vi "RunTest.vi"(8 "error in (no error)":errorcluster, 11 "Prueba10 in":refnum<class "Prueba10.lvclass">) -> (0 "error out":errorcluster, 2 "resultado":string, 3 "Prueba10 out":refnum<class "Prueba10.lvclass">)   [LabVIEW 2019, in "Prueba10.lvclass"]
uses:
  Prueba10.lvclass
  Prueba04/Control/Slide.ctl
  Prueba10.lvclass/Prueba10.ctl
  ClusterGEN.ctl
  <vilib>/Utility/error.llb/DialogType.ctl
  QMH/Message Queue/Enqueue Message (Single).vi
  <vilib>/Utility/error.llb/Error Cluster From Error Code.vi
  <vilib>/ErrorRing/Error Ring.xnode
  <vilib>/Utility/miscctls.llb/LVRowAndColumnTypeDef.ctl
  Prueba/Prueba.lvclass
  Controles/EstadosP10.ctl
  Controles/MessageP10.ctl
  QMH/User Event - Stop/User Event - Stop.lvlib
  QMH/Message Queue/Message Queue.lvlib
  Prueba04/Prueba04.lvclass
panel:
  out "Pict Ring 2":u16(ring)
  out "Pict Ring 3":u16(ring)
  out "cumple_no_cumple":bool
  out "Vref":dbl
  in  "Tab":enum32{"Page 1", "Page 2"}(tab)
  out "NivMaxMenosSens":dbl
  out "NivelRMSensayo":dbl
  out "frecuencia1":dbl
  in  "guardar_Vref":bool
  in  "generar1":bool
  in  "AjusteAmp":T1=40.0 caption="Ajuste de amplitud [mV]" scale=0.0..20000.0
  out "voltMon1":dbl format="%#.1f"
  out "frecMon1":dbl format="%#.1f"
  in  "seguir":bool
  out "Pict Ring 4":u16(ring)
  out "Pict Ring":u16(ring)
  in  "Tabla2":string[][](table)
  out "saltoMon":dbl format="%#.1f"
  in  "generar2":bool
  in  "resta":bool
  in  "suma":bool
  in  "salto":dbl(knob)=0.5 min=0.1 max=0.5 scale=0.1..0.5
  in  "semiciclo":dbl(knob)=1.0 min=1.0 max=2.0 scale=1.0..2.0
  in  "Tabla1":string[][](table)
  in  "salir":bool
  out "cumple":bool
  out "no_cumple":bool
  out "voltMon2":dbl format="%#.1f"
  out "frecMon2":dbl format="%#.1f"
  # "Selección de Señal de referencia 8000 Hz"
  # "Elección Señal de Referencia\nsegún marca y modelo de sonómetro"
  # "Nivel RMS para Ensayo"
  # "Nivel Máximo Rango \nMenos Sensible"
  # "Frecuencia"
  # "Monitoreo"
  # "Frecuencia"
  # "Hz"
  # "Voltaje"
  # "mV"
  # "10. Indicación de sobrecarga. IEC 61672-3: 2006 Cláusula 18"
  # "Tabla Resultados"
  # "Selección de Saltos"
  # "Selección Orientación Semiciclo"
  # "Cumple"
  # "No Cumple"
  # "10. Indicación de sobrecarga. IEC 61672-3: 2006 Cláusula 18"
  # "Monitoreo"
  # "Frecuencia"
  # "Hz"
  # "Voltaje"
  # "mV"
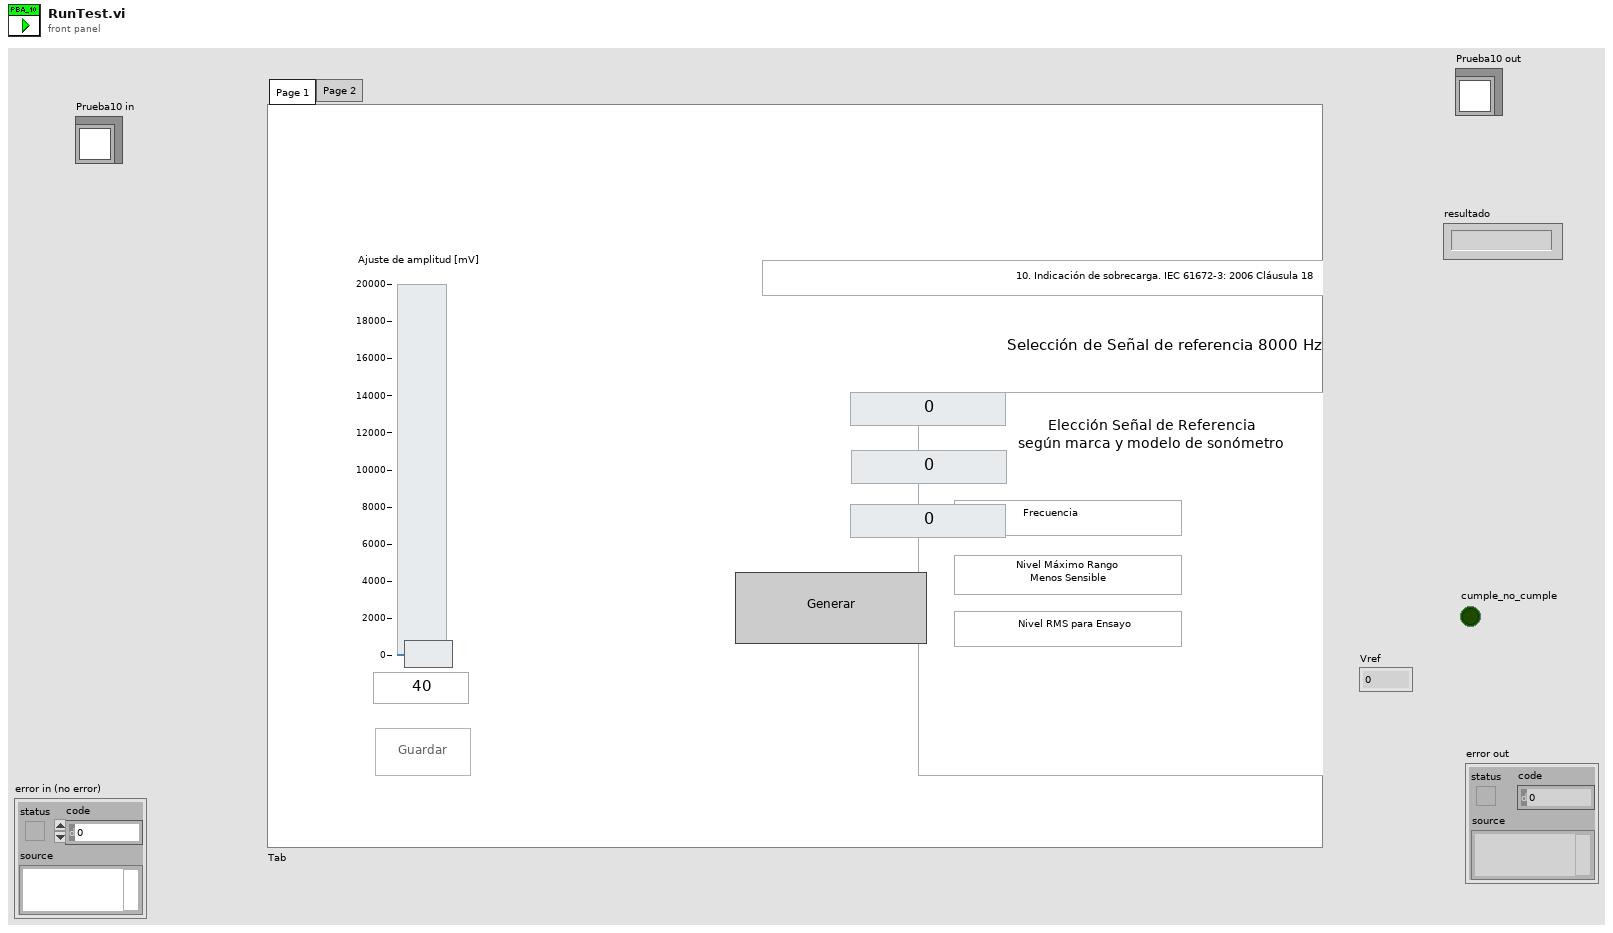
[diagram p1: front panel]
types:
  T1 = typedef "Prueba04.lvclass/Slide.ctl" = dbl
  T2 = typedef "LVRowAndColumnTypeDef.ctl" = cluster{"Row":i32, "Column":i32}
  T3 = typedef "Message Queue.lvlib/All Message Queues.ctl" = cluster{"MHL":refnum<queue>, "Inst_CNT90":refnum<queue>, "Inst_DS360":refnum<queue>, "Inst_Keithley2002":refnum<queue>, "Inst_DAQ":refnum<queue>, "BD":refnum<queue>, "Pistofono":refnum<queue>, "Nexus":refnum<queue>}
  T4 = enum32{"Page 1", "Page 2", "Page 3", "Page 4", "Page 5", "Page 6", "Page 7"}
  T5 = typedef "Prueba10.lvclass/ClusterGEN.ctl" = cluster{"frec":dbl, "amp":dbl}
  T6 = typedef "Prueba10.lvclass/EstadosP10.ctl" = enum16{"DetieneInstrumentos", "InicializarInstrumentos", "LeerArchivoConfiguracion", "Error", "inicio", "configurarTabla", "FrecAmp1", "FrecAmp2", "FrecAmp3", "suma_resta", "calcularVref", "iniciarGEN", "iniciarGEN_2", "reset-NivRefEnsayo", "guardaVref", "monitoreo", "monitoreo_2", "ingresaMediciones", "guardarMediciones", "detenerGEN", "cumplimiento", "listo_evaluar", "evaluar", "final", "salir"}
  T7 = typedef "Prueba10.lvclass/MessageP10.ctl" = cluster{"Estados":T6, "Data":variant}
  T8 = enum8{"Enabled", "Disabled", "Disabled and Grayed Out"}
  T9 = cluster{"ControlName":string, "ControlReference":refnum<vi>}[]
  T10 = typedef "DialogType.ctl" = u16
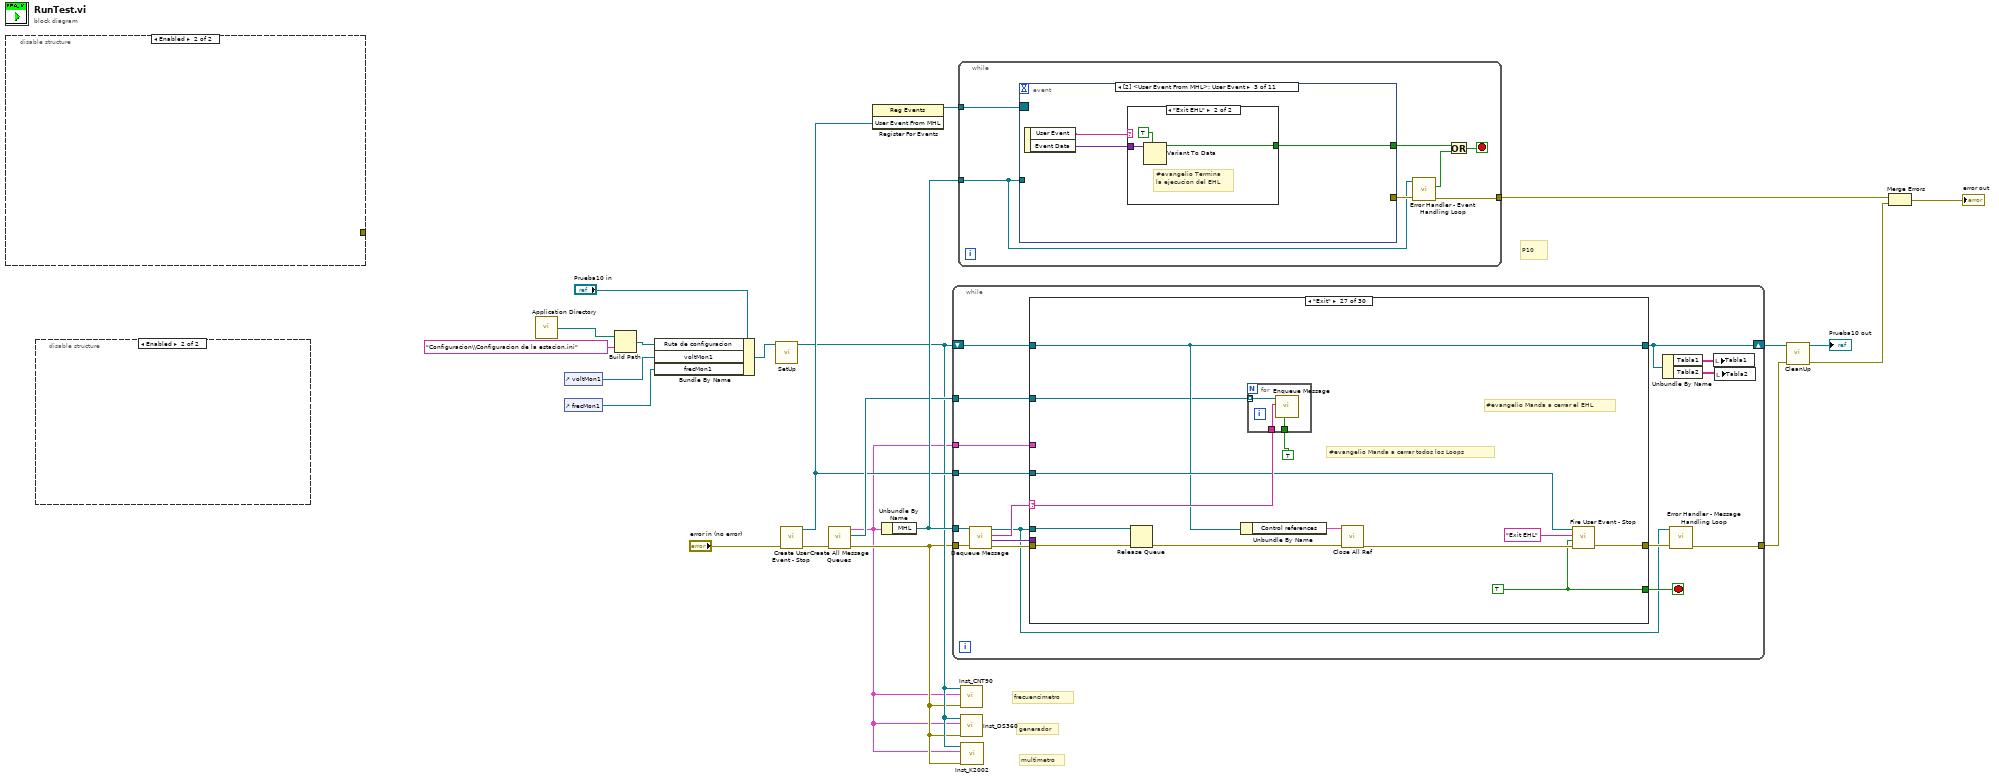
[diagram p0: block diagram]
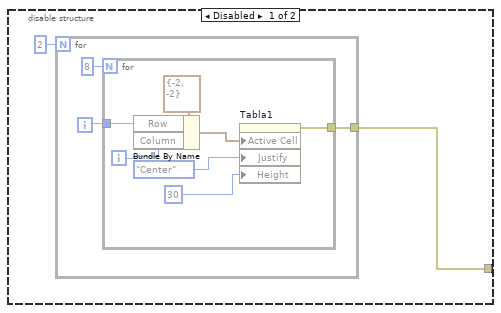
[diagram p2: hidden frame]
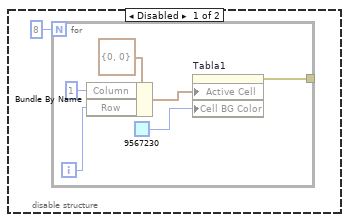
[diagram p3: hidden frame]
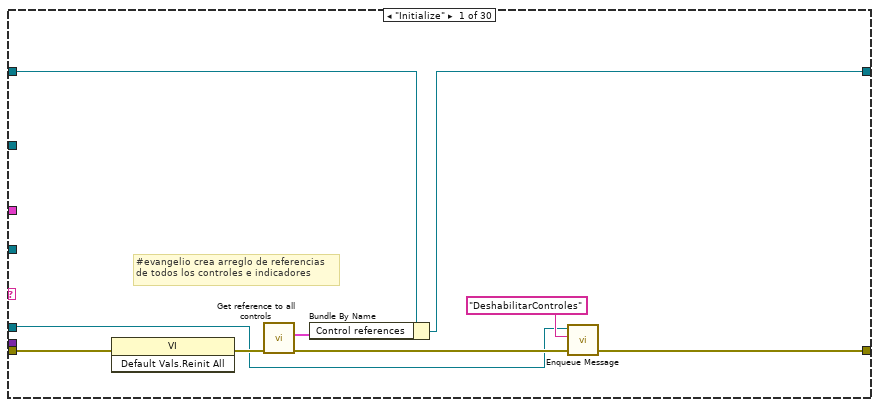
[diagram p4: hidden frame]
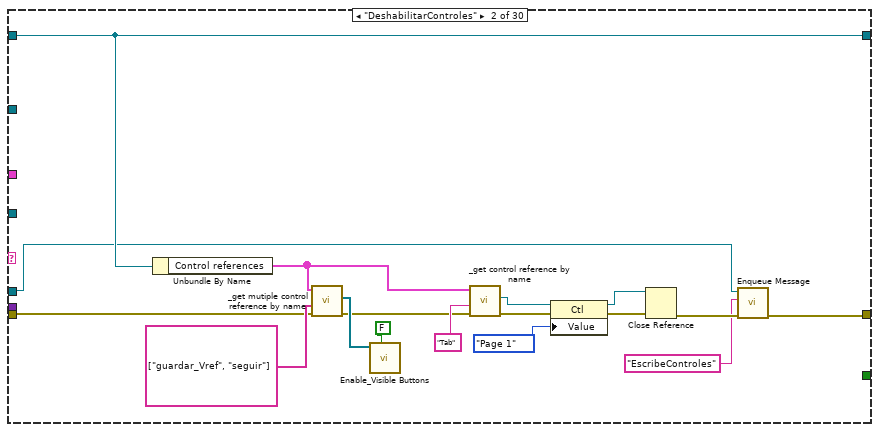
[diagram p5: hidden frame]
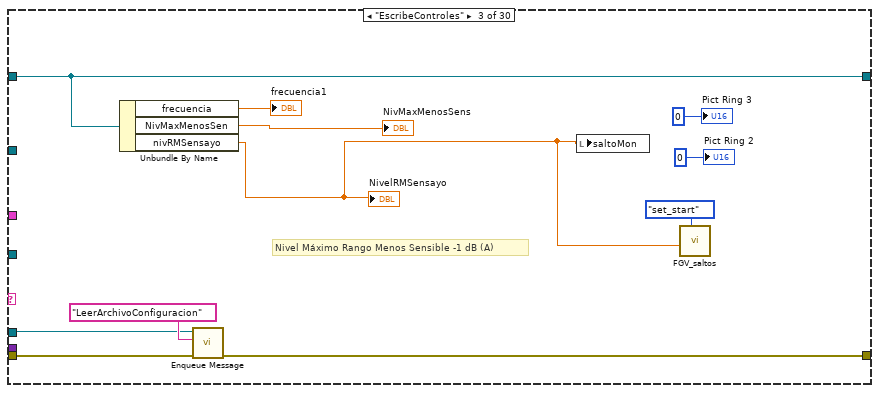
[diagram p6: hidden frame]
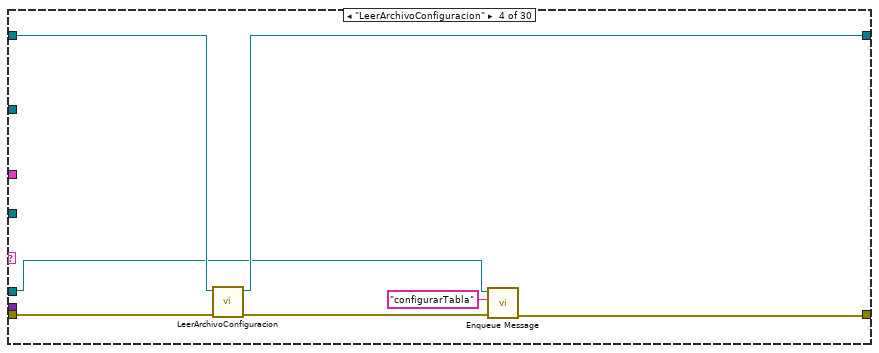
[diagram p7: hidden frame]
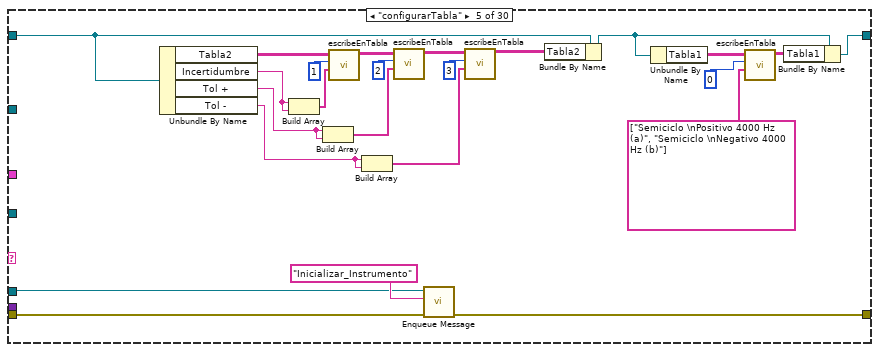
[diagram p8: hidden frame]
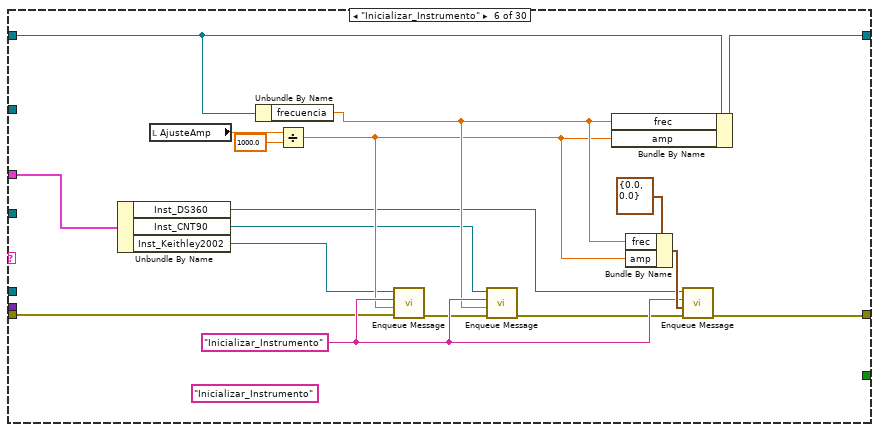
[diagram p9: hidden frame]
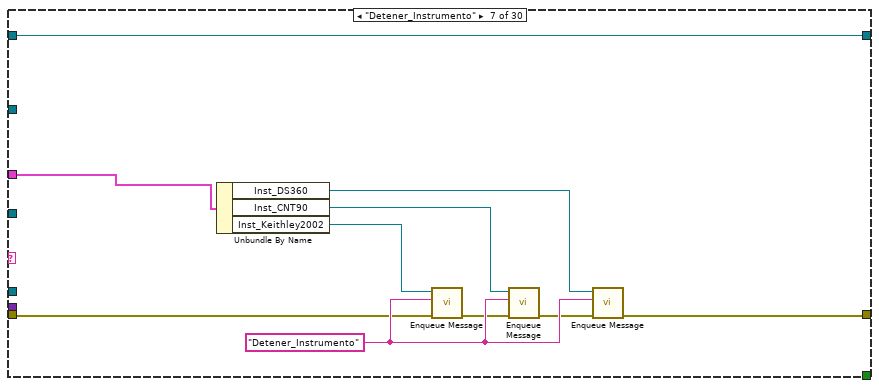
[diagram p10: hidden frame]
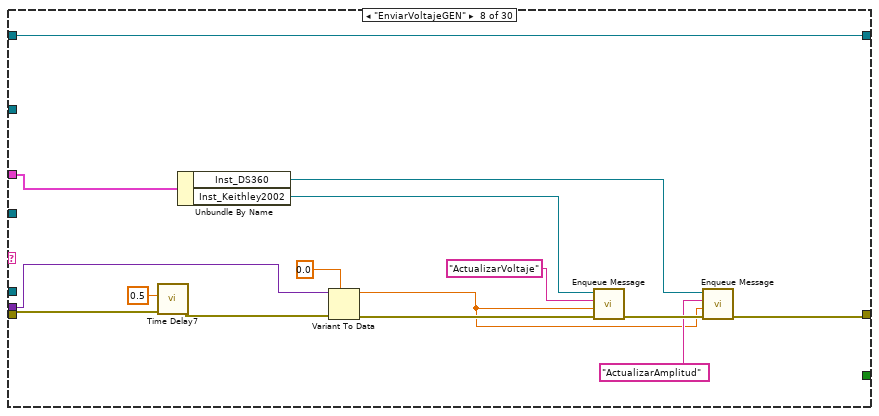
[diagram p11: hidden frame]
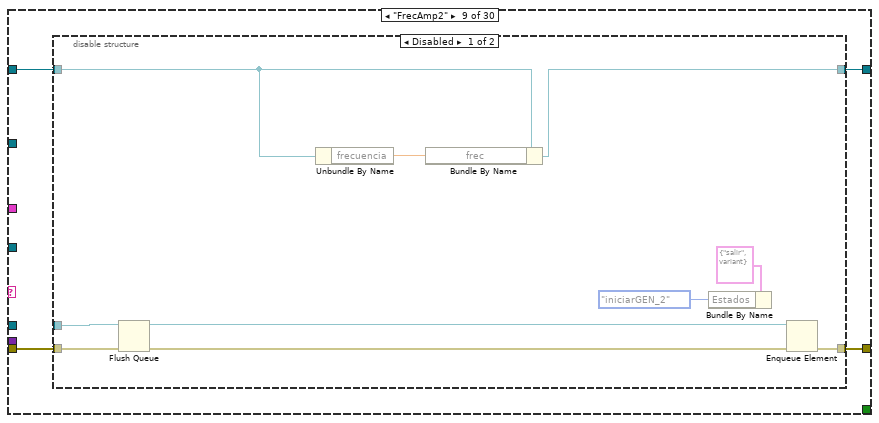
[diagram p12: hidden frame]
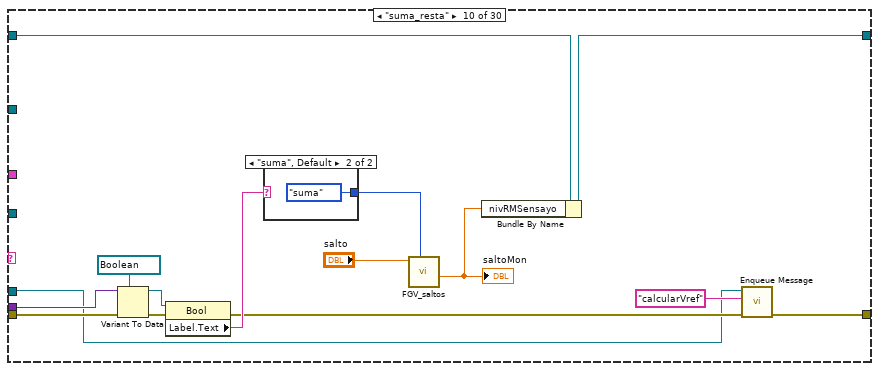
[diagram p14: hidden frame]
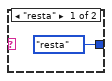
[diagram p15: hidden frame]
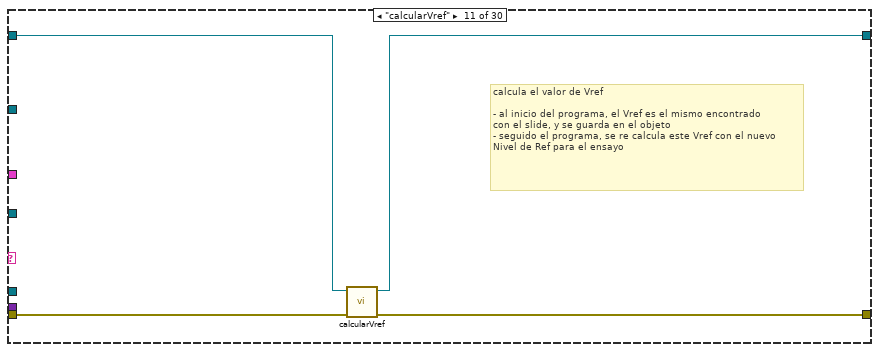
[diagram p16: hidden frame]
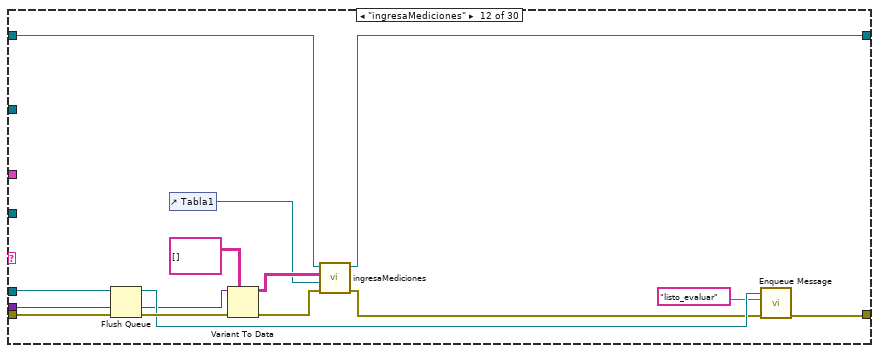
[diagram p17: hidden frame]
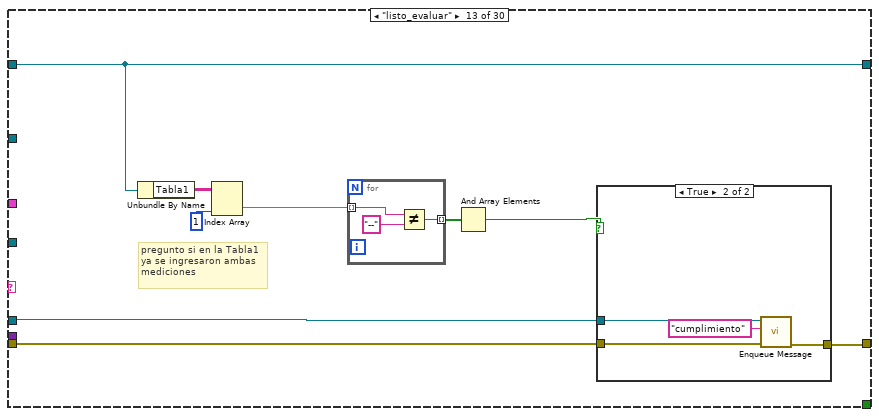
[diagram p18: hidden frame]
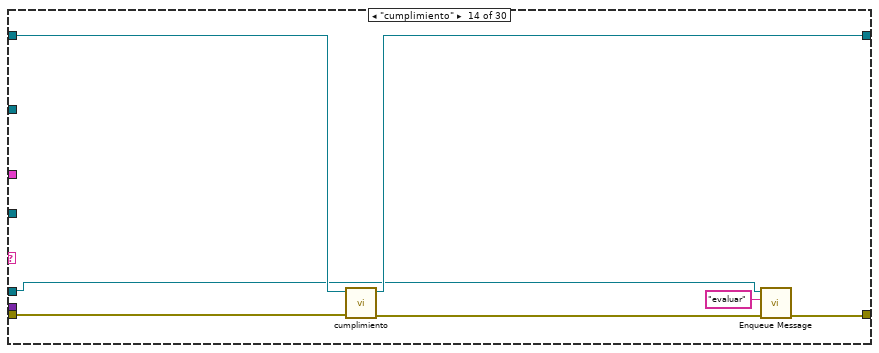
[diagram p20: hidden frame]
diagram:
  # "multimetro"
  # "generador"
  # "frecuencimetro"
  # "P10"
  n1 = disable-structure shown="Enabled" {
    disable-tunnel: [w24 _] -> _
    frame Disabled {
      n2 = for {
        N: 2 -> [_]
        tunnel: [w27] -> w24
        i -> [w26]
        n3 = for {
          N: 8 -> [_]
          tunnel: [w32] -> w27
          tunnel: w26 -> [w29]
          i -> [w28]
          n4 = Bundle By Name(cluster=T2 {"Row"=-2, "Column"=-2} ("Active Cell:Active Cell"), "Row"=w29, "Column"=w28) -> (w30:T2)
          n5 = property on="Tabla1" class="Tbl (strict)"("Active Cell"=w30, "Justify"=enum16{"Left", "Center", "Right"}."Center" ("Active Cell:Cell Justification"), "Height"=u32 30 ("Active Cell:Cell Font:Size")) -> (error out=w32:errorcluster)  [unwired: 2 in, 1 out]
        }
      }
    }
    frame Enabled {
    }
  }
  n6 = disable-structure shown="Enabled" {
    frame Disabled {
      n7 = for {
        N: 8 -> [_]
        tunnel: [w37] -> _
        i -> [w36]
        n8 = Bundle By Name(cluster=T2 {"Row"=0, "Column"=0} ("Active Cell:Active Cell"), "Column"=1, "Row"=w36) -> (w39:T2)
        n9 = property on="Tabla1" class="Tbl (strict)"("Active Cell"=w39, "Cell BG Color"=u32 9567230) -> (error out=w37:errorcluster)  [unwired: 2 in, 1 out]
      }
    }
    frame Enabled {
    }
  }
  n10 = call <vilib>:"Application Directory.vi"() -> ("Application Directory"=w19:path)
  n11 = control-ref of="voltMon1"() -> (w7:refnum<vi>)
  n12 = control-ref of="frecMon1"() -> (w6:refnum<vi>)
  n13 = Build Path(base path=w19, name or relative path="Configuracion\\Configuracion de la estacion.ini") -> (appended path=w18:path)
  n14 = Bundle By Name(cluster="Prueba10 in", "Ruta de configuracion"=w18, "voltMon1"=w7, "frecMon1"=w6) -> (w16:refnum<class "Prueba10.lvclass">)
  n15 = call-dynamic "SetUp.vi"("Prueba10 in"=w16) -> ("Prueba10 out"=w9:refnum<class "Prueba10.lvclass">)  [unwired: 9 in, 1 out]
  n16 = call "Create User Event - Stop.vi"("error in (no error)"="error in (no error)") -> ("error out"=w15:errorcluster, "User Event From MHL"=w10:refnum<user-event>)  [unwired: 9 in]
  n17 = call "Create All Message Queues.vi"("error in (no error)"=w15) -> ("error out"=w8:errorcluster, "PL Queues Array"=w11:refnum<queue>[], "All Message Queues out"=w5:T3)  [unwired: 8 in]
  n18 = register-events(w10) -> (reference out=w12:refnum<event-registration>)  [unwired: 2 in, 1 out]
  n19 = Unbundle By Name(w5) -> ("MHL"=w14:refnum<queue>)
  n20 = while {
    tunnel: w14 -> [w52]
    tunnel: w8 -> [w51]
    tunnel: [w47] -> w2
    shift-right: [w56] -> w4
    shift-left: w9 -> [w57]
    tunnel: w11 -> [w46]
    tunnel: w10 -> [w45]
    tunnel: w5 -> [w42]
    stop <- w53 stop-if-true
    n21 = call "Dequeue Message.vi"("error in (no error)"=w51, "Message Queue"=w52) -> ("error out"=w44:errorcluster, "Message Data"=w49:variant, "Message"=w50:string, "dup Message Queue"=w43:refnum<queue>)  [unwired: 6 in]
    n22 = case shown="\"Exit\"" w50 {
      selector: w50 -> [_ _ _ _ _ _ _ _ _ _ _ _ _ _ _ _ _ _ _ _ _ _ _ _ _ _ w405 _ w433 _]
      tunnel: w49 -> [_ _ _ _ _ _ _ w157 _ w193 _ w213 _ _ _ _ _ _ _ _ _ _ _ _ _ w391 _ _ _ _]
      tunnel: w44 -> [w62 w70 w94 w101 w120 w138 w145 w158 w171 w196 w204 w218 w227 w242 w251 w259 w266 w277 w290 w307 w321 w327 w351 w365 w389 w393 w408 w418 _ w442]
      tunnel: [w61 w68 w93 w97 w104 w135 w144 w156 w170 w186 w203 w217 w226 w240 w250 w259 w264 w276 w289 w306 w320 w325 w352 w365 w379 w392 w407 w417 w432 w442] -> w48
      tunnel: [_ _ _ _ _ _ _ _ _ _ _ _ _ _ _ _ _ _ _ _ _ _ _ _ _ _ w406 _ _ _] -> w53
      tunnel: w57 -> [w60 w69 w88 w100 w108 w142 w152 w167 w168 w198 w202 w207 w221 w238 w248 w254 w273 w286 w299 w305 w322 w326 w356 w375 w387 w399 w403 w423 w434 w443]
      tunnel: [w59 w69 w88 w99 w109 w141 w152 w167 w169 w188 w201 w211 w221 w239 w248 w254 w273 w286 w299 w305 w322 w326 w355 w366 w382 w399 w403 w423 w434 w443] -> w56
      tunnel: w46 -> [_ _ _ _ _ _ _ _ _ _ _ _ _ _ _ _ _ _ _ _ _ _ _ _ _ _ w402 _ _ _]
      tunnel: w45 -> [_ _ _ _ _ _ _ _ _ _ _ _ _ _ _ _ _ _ _ _ _ _ _ _ _ _ w404 _ _ _]
      tunnel: w43 -> [w58 w67 w84 w95 w102 _ _ _ _ w184 _ w205 w219 w236 w243 _ w262 w275 w288 w300 _ w324 _ _ w376 w390 w400 w416 _ _]
      tunnel: w42 -> [_ _ _ _ _ w127 w143 w153 _ _ _ _ _ _ _ _ w261 w274 w287 _ w313 w323 _ _ _ _ _ _ _ _]
      frame "Initialize" {
        # "#evangelio crea arreglo de referencias\nde todos los controles e indicadores"
        n23 = invoke class="VI" method="Default Vals.Reinit All"(error in=w62) -> (error out=w65:errorcluster)  [unwired: 2 in, 2 out]
        n24 = call "Get reference to all controls.vi"("error in (no error)"=w65) -> ("error out"=w63:errorcluster, "Control references"=w64:T9)  [unwired: 5 in]
        n25 = Bundle By Name(cluster=w60, "Control references"=w64) -> (w59:refnum<class "Prueba10.lvclass">)
        n26 = call-poly "Enqueue Message.vi"("error in (no error)"=w63, "Message"="DeshabilitarControles", "Message Queue"=w58) -> ("error out"=w61:errorcluster)  [unwired: 7 in, 1 out]
      }
      frame "DeshabilitarControles" {
        n27 = Unbundle By Name(w69) -> ("Control references"=w79:T9)
        n28 = call "_get mutiple control reference by name.vi"("error in (no error)"=w70, "Control names"=string[] ["guardar_Vref", "seguir"], "Control references"=w79) -> ("error out"=w76:errorcluster, "References"=w77:refnum<vi>[])  [unwired: 3 in]
        n29 = call "Enable_Visible Buttons.vi"("Enable? (T)"=FALSE, "Controls Ref Array"=w77) -> ()  [unwired: 10 in]
        n30 = call "_get control reference by name.vi"("error in (no error)"=w76, "Control name"="Tab" ("Message"), "Control references"=w79) -> ("error out"=w83:errorcluster, "Ctl Refnum"=w81:refnum<vi>)  [unwired: 3 in]
        n31 = property class="Ctl"(reference=w81, error in=w83, "Value"=T4."Page 1" ("Tab_Prueba04")) -> (reference out=w72:refnum<vi>, error out=w74:errorcluster)
        n32 = Close Reference(reference=w72, error in (no error)=w74) -> (error out=w73:errorcluster)
        n33 = call-poly "Enqueue Message.vi"("error in (no error)"=w73, "Message"="EscribeControles", "Message Queue"=w67) -> ("error out"=w68:errorcluster)  [unwired: 7 in, 1 out]
      }
      frame "EscribeControles" {
        # "Nivel Máximo Rango Menos Sensible -1 dB (A)"
        n34 = Unbundle By Name(w88) -> ("frecuencia"=→"frecuencia1":dbl, "NivMaxMenosSen"=→"NivMaxMenosSens":dbl, "nivRMSensayo"=w86:dbl)
        "NivelRMSensayo" <- w86
        n35 = call-poly "Enqueue Message.vi"("error in (no error)"=w94, "Message"="LeerArchivoConfiguracion", "Message Queue"=w84) -> ("error out"=w93:errorcluster)  [unwired: 7 in, 1 out]
        n36 = local write "saltoMon"(w86) -> ()
        n37 = call "FGV_saltos.vi"("action"=enum16{"suma", "resta", "set_start", "get"}."set_start", "NivRef in in"=w86) -> ()  [unwired: 8 in, 2 out]
        "Pict Ring 2" <- u16 0 ("Pict Ring 2")
        "Pict Ring 3" <- u16 0 ("Pict Ring 3")
      }
      frame "LeerArchivoConfiguracion" {
        n38 = call "LeerArchivoConfiguracion.vi"("error in"=w101, "Prueba10 in"=w100) -> ("error out"=w98:errorcluster, "Prueba10 out"=w99:refnum<class "Prueba10.lvclass">)  [unwired: 8 in]
        n39 = call-poly "Enqueue Message.vi"("error in (no error)"=w98, "Message"="configurarTabla", "Message Queue"=w95) -> ("error out"=w97:errorcluster)  [unwired: 7 in, 1 out]
      }
      frame "configurarTabla" {
        n40 = Unbundle By Name(w108) -> ("Tabla2"=w116:string[][], "Incertidumbre"=w115:string, "Tol +"=w113:string, "Tol -"=w111:string)
        n41 = Build Array(w115, w115) -> (w114:string[])
        n42 = Build Array(w113, w113) -> (w112:string[])
        n43 = call "escribeEnTabla.vi"("parametros"=w114, "col"=1, "tabla in"=w116) -> ("tabla out"=w125:string[][])  [unwired: 8 in]
        n44 = Build Array(w111, w111) -> (w110:string[])
        n45 = call "escribeEnTabla.vi"("parametros"=w112, "col"=2, "tabla in"=w125) -> ("tabla out"=w124:string[][])  [unwired: 8 in]
        n46 = call-poly "Enqueue Message.vi"("error in (no error)"=w120, "Message"="Inicializar_Instrumento", "Message Queue"=w102) -> ("error out"=w104:errorcluster)  [unwired: 7 in, 1 out]
        n47 = call "escribeEnTabla.vi"("parametros"=w110, "col"=3, "tabla in"=w124) -> ("tabla out"=w105:string[][])  [unwired: 8 in]
        n48 = Bundle By Name(cluster=w108, "Tabla2"=w105) -> (w106:refnum<class "Prueba10.lvclass">)
        n49 = Unbundle By Name(w106) -> ("Tabla1"=w107:string[][])
        n50 = call "escribeEnTabla.vi"("parametros"=string[] ["Semiciclo \nPositivo 4000 Hz (a)", "Semiciclo \nNegativo 4000 Hz (b)"], "col"=0, "tabla in"=w107) -> ("tabla out"=w119:string[][])  [unwired: 8 in]
        n51 = Bundle By Name(cluster=w106, "Tabla1"=w119) -> (w109:refnum<class "Prueba10.lvclass">)
      }
      frame "Inicializar_Instrumento" {
        (unwired) "Inicializar_Instrumento" ("Message")
        w139 = "Inicializar_Instrumento" ("Message")
        n52 = Unbundle By Name(w127) -> ("Inst_DS360"=w128:refnum<queue>, "Inst_CNT90"=w129:refnum<queue>, "Inst_Keithley2002"=w126:refnum<queue>)
        n53 = local read "AjusteAmp"() -> (w134:T1)
        n54 = Unbundle By Name(w142) -> ("frecuencia"=w136:dbl)
        n55 = Divide(x=w134, y=T1 1000.0) -> (x/y=w130:T1)
        n56 = call-poly "Enqueue Message.vi"("error in (no error)"=w138, "Message Data"=w130, "Message"=w139, "Message Queue"=w126) -> ("error out"=w132:errorcluster)  [unwired: 6 in, 1 out]
        n57 = call-poly "Enqueue Message.vi"("error in (no error)"=w132, "Message Data"=w136, "Message"=w139, "Message Queue"=w129) -> ("error out"=w131:errorcluster)  [unwired: 6 in, 1 out]
        n58 = Bundle By Name(cluster=w142, "frec"=w136, "amp"=w130) -> (w141:refnum<class "Prueba10.lvclass">)
        n59 = Bundle By Name(cluster=T5 {"frec"=0.0, "amp"=0.0} ("clusterGEN"), "frec"=w136, "amp"=w130) -> (w140:T5)
        n60 = call-poly "Enqueue Message.vi"("error in (no error)"=w131, "Message Data"=w140, "Message"=w139, "Message Queue"=w128) -> ("error out"=w135:errorcluster)  [unwired: 6 in, 1 out]
      }
      frame "Detener_Instrumento" {
        w148 = "Detener_Instrumento" ("Message")
        n61 = Unbundle By Name(w143) -> ("Inst_DS360"=w151:refnum<queue>, "Inst_CNT90"=w150:refnum<queue>, "Inst_Keithley2002"=w149:refnum<queue>)
        n62 = call-poly "Enqueue Message.vi"("error in (no error)"=w145, "Message"=w148, "Message Queue"=w149) -> ("error out"=w147:errorcluster)  [unwired: 7 in, 1 out]
        n63 = call-poly "Enqueue Message.vi"("error in (no error)"=w147, "Message"=w148, "Message Queue"=w150) -> ("error out"=w146:errorcluster)  [unwired: 7 in, 1 out]
        n64 = call-poly "Enqueue Message.vi"("error in (no error)"=w146, "Message"=w148, "Message Queue"=w151) -> ("error out"=w144:errorcluster)  [unwired: 7 in, 1 out]
      }
      frame "EnviarVoltajeGEN" {
        n65 = call "Time Delay7"("error in (no error)"=w158, "Delay Time (s)"=0.5) -> ("error out"=w155:errorcluster)  [unwired: 9 in]
        n66 = Unbundle By Name(w153) -> ("Inst_DS360"=w161:refnum<queue>, "Inst_Keithley2002"=w166:refnum<queue>)
        n67 = Variant To Data(error in=w155, type=0.0, Variant=w157) -> (data=w159:dbl, error out=w164:errorcluster)
        n68 = call-poly "Enqueue Message.vi"("error in (no error)"=w164, "Message Data"=w159, "Message"="ActualizarVoltaje", "Message Queue"=w166) -> ("error out"=w162:errorcluster)  [unwired: 6 in, 1 out]
        n69 = call-poly "Enqueue Message.vi"("error in (no error)"=w162, "Message Data"=w159, "Message"="ActualizarAmplitud", "Message Queue"=w161) -> ("error out"=w156:errorcluster)  [unwired: 6 in, 1 out]
      }
      frame "FrecAmp2" {
        n70 = disable-structure shown="Disabled" {
          disable-tunnel: w171 -> [w181 w182]
          disable-tunnel: [w180 w182] -> w170
          disable-tunnel: _ -> [w178 _]
          disable-tunnel: [w174 w183] -> w169
          disable-tunnel: w168 -> [w173 w183]
          frame Disabled {
            n71 = Flush Queue(queue=w178, error in (no error)=w181) -> (queue out=w177:refnum<queue>, error out=w179:errorcluster)  [unwired: 1 out]
            n72 = Unbundle By Name(w173) -> ("frecuencia"=w175:dbl)
            n73 = Bundle By Name(cluster=w173, "frec"=w175) -> (w174:refnum<class "Prueba10.lvclass">)
            n74 = Bundle By Name(cluster=T7 {"Estados"=enum."salir", "Data"=variant} ("MessageP08"), "Estados"=EstadosP10."iniciarGEN_2") -> ()  [unwired: 1 out]
            n75 = Enqueue Element(queue=w177, error in (no error)=w179) -> (error out=w180:errorcluster)  [unwired: 2 in, 2 out]
          }
          frame Enabled {
          }
        }
      }
      frame "suma_resta" {
        n76 = Variant To Data(error in=w196, type=refnum<vi> refnum ("CtlRef"), Variant=w193) -> (data=w191:refnum<vi>, error out=w194:errorcluster)
        n77 = property class="Bool"(reference=w191, error in=w194) -> (error out=w195:errorcluster, "Label.Text"=w197:string)  [unwired: 1 out]
        n78 = case shown="\"suma\", Default" w197 {
          tunnel: [enum16{"suma", "resta", "set_start", "get"}."resta" ("action") enum16{"suma", "resta", "set_start", "get"}."suma" ("action")] -> w190
          frame "resta" {
          }
          frame "suma", Default {
          }
        }
        n79 = call "FGV_saltos.vi"("action"=w190, "valor del salto"="salto") -> ("NivRef out"=w187:dbl)  [unwired: 8 in, 1 out]
        "saltoMon" <- w187
        n80 = Bundle By Name(cluster=w198, "nivRMSensayo"=w187) -> (w188:refnum<class "Prueba10.lvclass">)
        n81 = call-poly "Enqueue Message.vi"("error in (no error)"=w195, "Message"="calcularVref", "Message Queue"=w184) -> ("error out"=w186:errorcluster)  [unwired: 7 in, 1 out]
      }
      frame "calcularVref" {
        # "calcula el valor de Vref\n\n- al inicio del programa, el Vref es el mismo encontrado\ncon el slide, y se guarda en el objeto\n- seguido el programa, se re calcula este Vref con el nuevo \nNivel de Ref para el ensayo"
        n82 = call "calcularVref.vi"("error in (no error)"=w204, "Prueba10 in"=w202) -> ("error out"=w203:errorcluster, "Prueba10 out"=w201:refnum<class "Prueba10.lvclass">)  [unwired: 8 in]
      }
      frame "ingresaMediciones" {
        n83 = Flush Queue(queue=w205, error in (no error)=w218) -> (queue out=w215:refnum<queue>, error out=w216:errorcluster)  [unwired: 1 out]
        n84 = control-ref of="Tabla1"() -> (w209:refnum<vi>)
        n85 = Variant To Data(error in=w216, type=string[][] [] ("NewVal"), Variant=w213) -> (data=w210:string[][], error out=w212:errorcluster)
        n86 = call "ingresaMediciones.vi"("error in (no error)"=w212, "Tbl Refnum"=w209, "New Value"=w210, "Prueba09 in"=w207) -> ("error out"=w208:errorcluster, "Prueba09 out"=w211:refnum<class "Prueba10.lvclass">)  [unwired: 6 in]
        n87 = call-poly "Enqueue Message.vi"("error in (no error)"=w208, "Message"="listo_evaluar", "Message Queue"=w215) -> ("error out"=w217:errorcluster)  [unwired: 7 in, 1 out]
      }
      frame "listo_evaluar" {
        # "pregunto si en la Tabla1\nya se ingresaron ambas\nmediciones"
        n88 = Unbundle By Name(w221) -> ("Tabla1"=w220:string[][])
        n89 = Index Array(array=w220, index (col)=1 ("disabled index (col)")) -> (element=w223:string[])  [unwired: 1 in]
        n90 = for {
          tunnel: [w235] -> w224 mode=indexing
          tunnel: w223 -> [w233] mode=indexing
          n91 = Not Equal?(x=w233, y="--") -> (x != y?=w235:bool)
        }
        n92 = And Array Elements(Boolean array=w224) -> (logical AND=w222:bool)
        n93 = case shown="True" w222 {
          tunnel: w227 -> [w228 w232]
          tunnel: [w228 w231] -> w226
          tunnel: w219 -> [_ w230]
          frame False {
          }
          frame True {
            n94 = call-poly "Enqueue Message.vi"("error in (no error)"=w232, "Message"="cumplimiento", "Message Queue"=w230) -> ("error out"=w231:errorcluster)  [unwired: 7 in, 1 out]
          }
        }
      }
      frame "cumplimiento" {
        n95 = call "cumplimiento.vi"("error in (no error)"=w242, "Prueba09 in"=w238) -> ("error out"=w241:errorcluster, "Prueba09 out"=w239:refnum<class "Prueba10.lvclass">)  [unwired: 8 in]
        n96 = call-poly "Enqueue Message.vi"("error in (no error)"=w241, "Message"="evaluar", "Message Queue"=w236) -> ("error out"=w240:errorcluster)  [unwired: 7 in, 1 out]
      }
      frame "evaluar" {
        # "col"
        # "fila"
        n97 = Unbundle By Name(w248) -> ("Tabla2"=w247:string[][])
        n98 = Index Array(array=w247, index (row)=0 ("disabled index (row)"), index (col)=4 ("disabled index (col)")) -> (element=w249:string)
        n99 = Equal?(x=w249, y="Cumple") -> (x = y?=→"cumple_no_cumple":bool)
        n100 = call-poly "Enqueue Message.vi"("error in (no error)"=w251, "Message"="evaluar", "Message Queue"=w243) -> ("error out"=w250:errorcluster)  [unwired: 7 in, 1 out]
      }
      frame "final" {
        n101 = local read "cumple_no_cumple"() -> (w255:bool)
        "cumple" <- w255
        n102 = Not(x=w255) -> (.not. x?=→"no_cumple":bool)
        n103 = Select(t="Cumple", s=w255, f="No Cumple") -> (s? t:f=→"resultado":string)
      }
      frame "iniciarGEN" {
        n104 = Unbundle By Name(w261) -> ("Inst_DS360"=w271:refnum<queue>)
        n105 = call-poly "Enqueue Message.vi"("error in (no error)"=w266, "Message"="Habilitar_Generador", "Message Queue"=w271) -> ("error out"=w269:errorcluster)  [unwired: 7 in, 1 out]
        n106 = call "Time Delay"("error in (no error)"=w269, "Delay Time (s)"=0.5) -> ("error out"=w268:errorcluster)  [unwired: 9 in]
        n107 = call-poly "Enqueue Message.vi"("error in (no error)"=w268, "Message"="Leer_Voltaje", "Message Queue"=w262) -> ("error out"=w265:errorcluster)  [unwired: 7 in, 1 out]
        n108 = property on="guardar_Vref" class="Bool"(error in=w265, "DisabledEnum"=T8."Enabled" ("Disabled")) -> (error out=w264:errorcluster)  [unwired: 1 in, 1 out]
      }
      frame "Leer_Voltaje" {
        n109 = Flush Queue(queue=w275, error in (no error)=w277) -> (queue out=w278:refnum<queue>, error out=w279:errorcluster)  [unwired: 1 out]
        n110 = Unbundle By Name(w274) -> ("Inst_Keithley2002"=w282:refnum<queue>)
        n111 = call-poly "Enqueue Message.vi"("error in (no error)"=w279, "Message"="Leer_Frecuencia", "Message Queue"=w278) -> ("error out"=w285:errorcluster)  [unwired: 7 in, 1 out]
        n112 = call-poly "Enqueue Message.vi"("error in (no error)"=w285, "Message"="Leer_Instrumento", "Message Queue"=w282) -> ("error out"=w283:errorcluster)  [unwired: 7 in, 1 out]
        n113 = call "Time Delay2"("error in (no error)"=w283, "Delay Time (s)"=1.0) -> ("error out"=w276:errorcluster)  [unwired: 9 in]
      }
      frame "Leer_Frecuencia" {
        n114 = Flush Queue(queue=w288, error in (no error)=w290) -> (queue out=w291:refnum<queue>, error out=w292:errorcluster)  [unwired: 1 out]
        n115 = Unbundle By Name(w287) -> ("Inst_CNT90"=w295:refnum<queue>)
        n116 = call-poly "Enqueue Message.vi"("error in (no error)"=w292, "Message"="Leer_Indicadores", "Message Queue"=w291) -> ("error out"=w298:errorcluster)  [unwired: 7 in, 1 out]
        n117 = call-poly "Enqueue Message.vi"("error in (no error)"=w298, "Message"="Leer_Instrumento", "Message Queue"=w295) -> ("error out"=w296:errorcluster)  [unwired: 7 in, 1 out]
        n118 = call "Time Delay3"("error in (no error)"=w296, "Delay Time (s)"=1.0) -> ("error out"=w289:errorcluster)  [unwired: 9 in]
      }
      frame "Leer_Indicadores" {
        n119 = Flush Queue(queue=w300, error in (no error)=w307) -> (queue out=w308:refnum<queue>, error out=w309:errorcluster)  [unwired: 1 out]
        n120 = Unbundle By Name(w305) -> ("voltMon1"=w304:refnum<vi>, "frecMon1"=w303:refnum<vi>)
        n121 = property class="DigNum (strict)"(reference=w304) -> ("Value"=→"voltMon1" →"voltMon2":dbl)  [unwired: 1 in, 2 out]
        n122 = property class="DigNum (strict)"(reference=w303) -> ("Value"=→"frecMon1" →"frecMon2":dbl)  [unwired: 1 in, 2 out]
        n123 = call-poly "Enqueue Message.vi"("error in (no error)"=w309, "Message"="Leer_Voltaje", "Message Queue"=w308) -> ("error out"=w312:errorcluster)  [unwired: 7 in, 1 out]
        n124 = call "Time Delay4"("error in (no error)"=w312, "Delay Time (s)"=1.0) -> ("error out"=w306:errorcluster)  [unwired: 9 in]
      }
      frame "iniciarGEN_2" {
        w317 = T5 {"frec"=0.0, "amp"=0.0}  # clusterGEN
        # "Prepara la frec y amplitud para comenzar\nla generacion de la señal"
        n125 = Unbundle By Name(w322) -> ("frec"=w316:dbl, "amp"=w315:dbl)
        n126 = Unbundle By Name(w313) -> ("Inst_DS360"=w319:refnum<queue>)
        n127 = Bundle By Name(cluster=w317, "frec"=w316, "amp"=w315) -> (w314:T5)
        n128 = call-poly "Enqueue Message.vi"("error in (no error)"=w321, "Message Data"=w314, "Message"="iniciaGEN_Peak", "Message Queue"=w319) -> ("error out"=w320:errorcluster)  [unwired: 6 in, 1 out]
      }
      frame "detenerGEN" {
        w342 = 0.0 ("voltaje1")
        n129 = Flush Queue(queue=w324, error in (no error)=w327) -> (error out=w331:errorcluster)  [unwired: 2 out]
        n130 = Unbundle By Name(w323) -> ("Inst_DS360"=w336:refnum<queue>)
        n131 = call "Time Delay6"("error in (no error)"=w331, "Delay Time (s)"=0.5) -> ("error out"=w330:errorcluster)  [unwired: 9 in]
        n132 = call-poly "Enqueue Message.vi"("error in (no error)"=w330, "Message"="Deshabilitar_Generador", "Message Queue"=w336) -> ("error out"=w335:errorcluster)  [unwired: 7 in, 1 out]
        n133 = call "Time Delay5"("error in (no error)"=w335, "Delay Time (s)"=0.5) -> ("error out"=w334:errorcluster)  [unwired: 9 in]
        n134 = Unbundle By Name(w326) -> ("Control references"=w328:T9)
        n135 = call-poly "get control reference by name.vi"("error in (no error)"=w334, "Control name"="guardar_Vref" ("String"), "Control references"=w328) -> ("error out"=w329:errorcluster, "Ctl Refnum"=w339:refnum<vi>)  [unwired: 3 in]
        n136 = Build Array(w339) -> (w338:refnum<vi>[])
        n137 = call "Enable_Visible Buttons.vi"("Enable? (T)"=FALSE, "Controls Ref Array"=w338) -> ()  [unwired: 10 in]
        n138 = disable-structure shown="Enabled" {
          disable-tunnel: w329 -> [w345 w349]
          disable-tunnel: w328 -> [w344 _]
          disable-tunnel: [w343 w349] -> w325
          frame Disabled {
            n139 = call "_get mutiple control reference by name.vi"("error in (no error)"=w345, "Control names"=string[] ["genera3", "knobFrec"] ("tipo_ciclo"), "Control references"=w344) -> ("error out"=w343:errorcluster, "References"=w346:refnum<vi>[])  [unwired: 3 in]
            n140 = call "Enable_Visible Buttons.vi"("Enable? (T)"=TRUE, "Controls Ref Array"=w346) -> ()  [unwired: 10 in]
          }
          frame Enabled {
          }
        }
        n141 = local write "frecMon2"(w342) -> ()
        n142 = local write "voltMon2"(w342) -> ()
        n143 = local write "frecMon1"(w342) -> ()
        n144 = local write "voltMon1"(w342) -> ()
      }
      frame "guardaVref" {
        n145 = flat-sequence {
          tunnel: [w357] -> w354
          tunnel: w351 -> [w360]
          tunnel: [w360] -> w350
          frame #0 {
            n146 = local read "AjusteAmp"() -> (w359:T1)
            n147 = Divide(x=w359, y=T1 1000.0) -> (x/y=w357:T1)
            "Vref" <- w357
            n148 = Number To Fractional String(number=w359, precision (6)=i16 1) -> (F-format string=w361:string)  [unwired: 2 in]
            n149 = Format Into String(format string="Se guardó Vref = %s mV", w361) -> (resulting string=w364:string)  [unwired: 2 in, 1 out]
            n150 = One Button Dialog(message=w364) -> ()  [unwired: 1 in, 1 out]
          }
        }
        n151 = Bundle By Name(cluster=w356, "Vref"=w354) -> (w355:refnum<class "Prueba10.lvclass">)
        n152 = property on="seguir" class="Bool"(error in=w350, "DisabledEnum"=T8."Enabled" ("Disabled")) -> (error out=w352:errorcluster)  [unwired: 1 in, 1 out]
      }
      frame "guardarMediciones" {
        # "Guarda el Valor medido en DMM\nen la Tabla"
        n153 = Unbundle By Name(w375) -> ("Tabla1"=w374:string[][], "voltMedido"=w372:dbl)
        n154 = local read "semiciclo"() -> (w371:dbl)
        n155 = To Long Integer(number=w371) -> (32bit integer=w370:i32)
        n156 = Decrement(x=w370) -> (x-1=w369:i32)
        n157 = call "escribeEnTablaUnValor.vi"("element"=w372, "fila"=w369, "col"=2, "tabla in"=w374) -> ("tabla out"=w368:string[][])  [unwired: 7 in]
        n158 = Bundle By Name(cluster=w375, "Tabla1"=w368) -> (w366:refnum<class "Prueba10.lvclass">)
        n159 = Unbundle By Name(w366) -> ("Tabla1"=w367:string[][])
        n160 = local write "Tabla1"(w367) -> ()
      }
      frame "reset-NivRefEnsayo" {
        w378 = 0.5 items=["0,1 dB (A)"=0.1, "0,5 dB (A)"=0.5] ("salto")
        n161 = call-poly "Enqueue Message.vi"("error in (no error)"=w389, "Message"="calcularVref", "Message Queue"=w376) -> ("error out"=w383:errorcluster)  [unwired: 7 in, 1 out]
        n162 = Unbundle By Name(w387) -> ("NivMaxMenosSen"=w385:dbl)
        n163 = Subtract(x=w385, y=1.0) -> (x-y=w381:dbl)
        n164 = Bundle By Name(cluster=w387, "nivRMSensayo"=w381) -> (w382:refnum<class "Prueba10.lvclass">)
        n165 = call "FGV_saltos.vi"("action"=enum16{"suma", "resta", "set_start", "get"}."set_start", "error in (no error)"=w383, "NivRef in in"=w381) -> ("error out"=w380:errorcluster, "NivRef out"=w386:dbl)  [unwired: 7 in]
        n166 = local write "saltoMon"(w386) -> ()
        n167 = property on="salto" class="Knob (strict)"(error in=w380, "Value"=w378) -> (error out=w379:errorcluster)  [unwired: 1 in, 1 out]
      }
      frame "Error" {
        w397 = T10 1 items=["no dialog", "OK message", "continue or stop message", "OK message + warnings", "continue/stop + warnings"] ("type of dialog (OK msg:1)")
        n168 = Variant To Data(error in=w393, type=errorcluster {"status"=FALSE, "code"=0, "source"=""} ("error out"), Variant=w391) -> (data=w395:errorcluster, error out=w394:errorcluster)
        n169 = call <vilib>:"Simple Error Handler.vi"("type of dialog (OK msg:1)"=w397, "error in (no error)"=w395) -> ()  [unwired: 3 in, 5 out]
        n170 = call-poly "Enqueue Message.vi"("error in (no error)"=w394, "Message"="Exit", "Message Queue"=w390) -> ("error out"=w392:errorcluster)  [unwired: 7 in, 1 out]
      }
      frame "Exit" {
        w406 = TRUE
        # "#evangelio Manda a cerrar el EHL"
        # "#evangelio Manda a cerrar todos los Loops"
        n171 = Release Queue(queue=w400, error in (no error)=w408) -> (error out=w412:errorcluster)  [unwired: 1 in, 2 out]
        n172 = Unbundle By Name(w403) -> ("Control references"=w401:T9)
        n173 = for {
          tunnel: w405 -> [w415]
          tunnel: TRUE -> [w414]
          tunnel: w402 -> [w413] mode=indexing
          n174 = call-poly "Enqueue Message.vi"("Priority Message? (F)"=w414, "Message"=w415, "Message Queue"=w413) -> ()  [unwired: 7 in, 2 out]
        }
        n175 = call "Close All Ref.vi"("error in (no error)"=w412, "Control references"=w401) -> ("error out"=w410:errorcluster)  [unwired: 9 in]
        n176 = call "Fire User Event - Stop.vi"("error in (no error)"=w410, "Event Data"=w406, "User Event"="Exit EHL", "User Event in"=w404) -> ("error out"=w407:errorcluster)  [unwired: 7 in]
      }
      frame "Confirmar Salida" {
        n177 = Two Button Dialog(message="¿Quieres cerrar la aplicación?", 1:"No" ("T button name (\"OK\")"), 2:"Si" ("T button name (\"OK\")")) -> (T button?=w419:bool)
        n178 = case shown="True" w419 {
          tunnel: w418 -> [w424 w427]
          tunnel: [w424 w431] -> w417
          tunnel: w416 -> [_ w429]
          frame False {
          }
          frame True {
            n179 = call-poly "Enqueue Message.vi"("error in (no error)"=w427, "Message"="Detener_Instrumento", "Message Queue"=w429) -> ("error out"=w426:errorcluster, "dup Message Queue"=w428:refnum<queue>)  [unwired: 7 in]
            n180 = call-poly "Enqueue Message.vi"("error in (no error)"=w426, "Message"="Exit", "Message Queue"=w428) -> ("error out"=w431:errorcluster)  [unwired: 7 in, 1 out]
          }
        }
      }
      frame Default {
        n181 = xnode "Error Ring"("parameter 0"=w433) -> ("error out"=w432:errorcluster)
      }
      frame "---------Controles---------" {
      }
    }
    n182 = Unbundle By Name(w56) -> ("Tabla1"=w55:string[][], "Tabla2"=w54:string[][])
    n183 = call "Error Handler - Message Handling Loop.vi"("error in (no error)"=w48, "Message Queue"=w43) -> ("dup error in"=w47:errorcluster)  [unwired: 8 in, 1 out]
    n184 = local write "Tabla1"(w55) -> ()
    n185 = local write "Tabla2"(w54) -> ()
  }
  n186 = while {
    tunnel: w14 -> [w446]
    tunnel: [w447] -> w22
    tunnel: w12 -> [w450]
    stop <- w449 stop-if-true
    n187 = event shown="[2] <User Event From MHL>: User Event" {
      selector: w450 -> [_ _ _ _ _ _ _ _ _ _ _]
      dyn-events: _ -> [_ _ _ _ _ _ _ _ _ _ _]
      timeout: _ -> [_ _ _ _ _ _ _ _ _ _ _]
      tunnel: w446 -> [w456 w462 _ w472 w475 w479 w485 w488 w496 w500 w502]
      tunnel: [w452 w463 _ w471 w476 w480 w482 w486 w495 w499 w503] -> w448
      tunnel: [_ _ w464 _ _ _ _ _ _ _ _] -> w444
      event "salir": Value Change {
        n188 = event-data() -> ()  [unwired: 1 in, 1 out]
        n189 = call-poly "Enqueue Message.vi"("Message"="Detener_Instrumento", "Message Queue"=w456) -> ("error out"=w453:errorcluster, "dup Message Queue"=w454:refnum<queue>)  [unwired: 8 in]
        n190 = call-poly "Enqueue Message.vi"("error in (no error)"=w453, "Message"="Exit", "Message Queue"=w454) -> ("error out"=w452:errorcluster)  [unwired: 7 in, 1 out]
      }
      event "generar1": Value Change {
        n191 = event-data() -> ("NewVal"=w461:bool)  [unwired: 1 in]
        n192 = Select(t="iniciarGEN", s=w461, f="detenerGEN") -> (s? t:f=w458:string)
        n193 = call-poly "Enqueue Message.vi"("Priority Message? (F)"=TRUE, "Message"=w458, "Message Queue"=w462) -> ("error out"=w463:errorcluster)  [unwired: 7 in, 1 out]
      }
      event User Event {
        n194 = event-data() -> ("User Event"=w466:string, "Event Data"=w465:variant)  [unwired: 1 in]
        n195 = case shown="\"Exit EHL\"" w466 {
          tunnel: w465 -> [_ w468]
          tunnel: [_ w467] -> w464
          frame Default {
          }
          frame "Exit EHL" {
            # "#evangelio Termina\nla ejecucion del EHL"
            n196 = Variant To Data(type=TRUE, Variant=w468) -> (data=w467:bool)  [unwired: 1 in, 1 out]
          }
        }
      }
      event Panel Close? {
        w470 = TRUE
        n197 = event-data() -> ()  [unwired: 1 in, 1 out]
        n198 = call-poly "Enqueue Message.vi"("Priority Message? (F)"=w470, "Message"="Confirmar Salida", "Message Queue"=w472) -> ("error out"=w471:errorcluster)  [unwired: 7 in, 1 out]
        n199 = event-data("Discard?"=w470) -> ()  [unwired: 1 in, 1 out]
      }
      event "generar2": Value Change {
        n200 = event-data() -> ()  [unwired: 1 in, 1 out]
        n201 = call-poly "Enqueue Message.vi"("Message"="iniciarGEN_2", "Message Queue"=w475) -> ("error out"=w476:errorcluster)  [unwired: 8 in, 1 out]
      }
      event "suma", "resta": Value Change {
        n202 = event-data() -> ("CtlRef"=w477:refnum<vi>)  [unwired: 1 in]
        n203 = call-poly "Enqueue Message.vi"("Message Data"=w477, "Message"="suma_resta", "Message Queue"=w479) -> ("error out"=w480:errorcluster)  [unwired: 7 in, 1 out]
      }
      event "seguir": Value Change {
        n204 = event-data() -> ()  [unwired: 1 in, 1 out]
        n205 = call-poly "Enqueue Message.vi"("Message"="calcularVref", "Message Queue"=w485) -> ("error out"=w483:errorcluster)  [unwired: 8 in, 1 out]
        n206 = property on="Tab" class="TabCtl (strict)"(error in=w483, "Value"=enum32{"Page 1", "Page 2"}."Page 2" ("Tab")) -> (error out=w482:errorcluster)  [unwired: 1 in, 1 out]
      }
      event Value Change {
        # "mV"
        n207 = event-data() -> ()  [unwired: 1 in, 1 out]
        n208 = Divide(x="AjusteAmp", y=T1 1000.0) -> (x/y=w490:T1)
        n209 = call-poly "Enqueue Message.vi"("Priority Message? (F)"=TRUE, "Message Data"=w490, "Message"="EnviarVoltajeGEN", "Message Queue"=w488) -> ("error out"=w486:errorcluster)  [unwired: 6 in, 1 out]
      }
      event "guardar_Vref": Value Change {
        n210 = event-data() -> ()  [unwired: 1 in, 1 out]
        n211 = call-poly "Enqueue Message.vi"("Priority Message? (F)"=TRUE, "Message"="guardaVref", "Message Queue"=w496) -> ("error out"=w495:errorcluster)  [unwired: 7 in, 1 out]
      }
      event "Tabla1": Value Change {
        n212 = event-data() -> ("NewVal"=w497:string[][])  [unwired: 1 in]
        n213 = call-poly "Enqueue Message.vi"("Message Data"=w497, "Message"="ingresaMediciones", "Message Queue"=w500) -> ("error out"=w499:errorcluster)  [unwired: 7 in, 1 out]
      }
      event "semiciclo": Value Change {
        n214 = event-data() -> ()  [unwired: 1 in, 1 out]
        n215 = call-poly "Enqueue Message.vi"("Message"="reset-NivRefEnsayo", "Message Queue"=w502) -> ("error out"=w503:errorcluster)  [unwired: 8 in, 1 out]
      }
    }
    n216 = call "Error Handler - Event Handling Loop.vi"("error in (no error)"=w448, "Message Queue"=w446) -> ("dup error in"=w447:errorcluster, "Error?"=w445:bool)  [unwired: 7 in, 1 out]
    n217 = Or(x=w444, y=w445) -> (x .or. y?=w449:bool)
  }
  n218 = call "Inst_CNT90.vi"("error in"=w8, "All Message Queues in"=w5, "Prueba31 in"=w9) -> ()  [unwired: 8 in, 1 out]
  n219 = call "Inst_DS360.vi"("error in"=w8, "All Message Queues in"=w5, "Prueba10 in"=w9) -> ()  [unwired: 8 in, 1 out]
  n220 = call "Inst_K2002.vi"("error in"=w8, "All Message Queues in"=w5, "Prueba31 in"=w9) -> ()  [unwired: 8 in, 1 out]
  n221 = call-dynamic "CleanUp.vi"("error in (no error)"=w2, "Prueba10 in"=w4) -> ("error out"=w1:errorcluster, "Prueba10 out"=→"Prueba10 out":refnum<class "Prueba10.lvclass">)  [unwired: 8 in]
  n222 = Merge Errors(w22, w1) -> (→"error out":errorcluster)
